vi "Get Unique ID.vi"(8 "error in (no error)":errorcluster, 11 "Step in":refnum<class "Step.lvclass">) -> (0 "error out":errorcluster, 2 "Unique ID":string, 3 "Step out":refnum<class "Step.lvclass">)   [LabVIEW 2020, in "TSnax.lvlib" / "Step.lvclass"]
uses:
  Step.lvclass
  Step.lvclass/Step.ctl
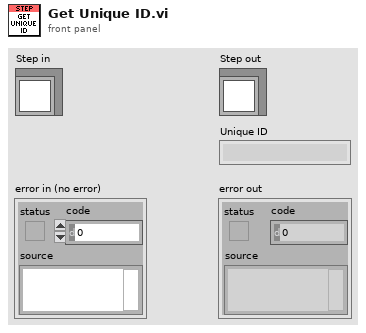
[diagram p1: front panel]
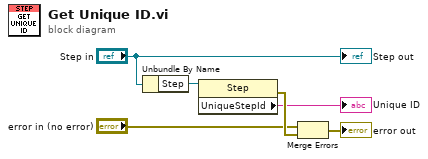
[diagram p0: block diagram]
diagram:
  n1 = Unbundle By Name("Step in") -> ("Step"=w3:refnum<k7>)
  n2 = property class="Step"(reference=w3) -> (error out=w6:errorcluster, "UniqueStepId"=→"Unique ID":string)  [unwired: 1 in, 1 out]
  n3 = Merge Errors("error in (no error)", w6) -> (→"error out":errorcluster)
  "Step out" <- "Step in"
